vi "Read frecuency.vi"(8 "error in (no error)":errorcluster, 11 "SignalIn in":refnum<class "SignalIn.lvclass">) -> (0 "error out":errorcluster, 2 "frecuency":dbl=1.0, 3 "SignalIn out":refnum<class "SignalIn.lvclass">)   [LabVIEW 2011, in "SignalIn.lvclass"]
uses:
  SignalIn.lvclass
  SignalIn.lvclass/SignalIn.ctl
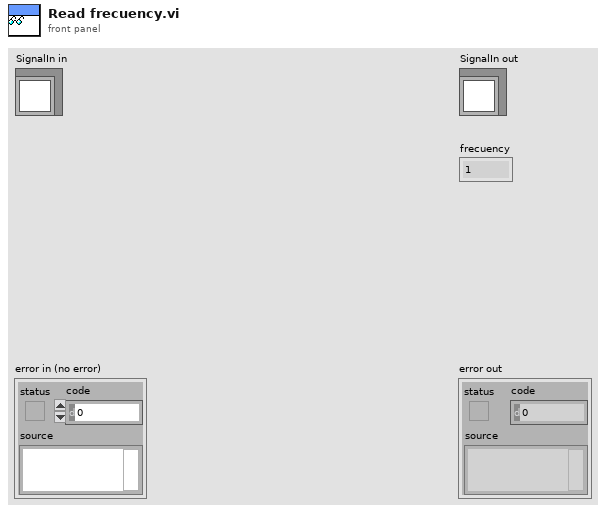
[diagram p1: front panel]
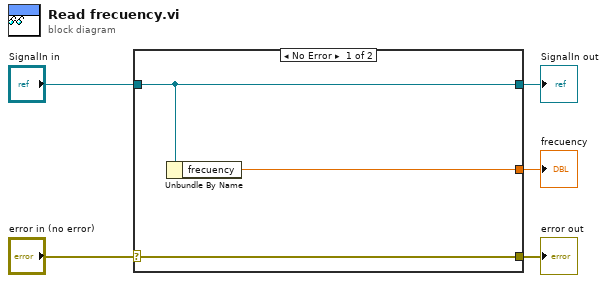
[diagram p0: block diagram]
diagram:
  n1 = case shown="No Error" "error in (no error)" {
    selector: "error in (no error)" -> [w8 w9]
    tunnel: [w8 w9] -> w4
    tunnel: [w7 w10] -> w2
    tunnel: "SignalIn in" -> [w7 w10]
    tunnel: [w6 _] -> w1
    frame No Error {
      n2 = Unbundle By Name(w7) -> ("frecuency"=w6:dbl)
    }
    frame Error {
    }
  }
  "error out" <- w4
  "SignalIn out" <- w2
  "frecuency" <- w1
